vi "Ejercicio 2.1.vi"() -> ()   [LabVIEW 2021]
panel:
  out "[0.75 , 1]":dbl
  out "[0.5 , 0.75]":dbl
  out "[0.25 , 0.5]":dbl
  out "[0 , 0.25]":dbl
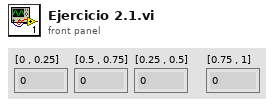
[diagram p1: front panel]
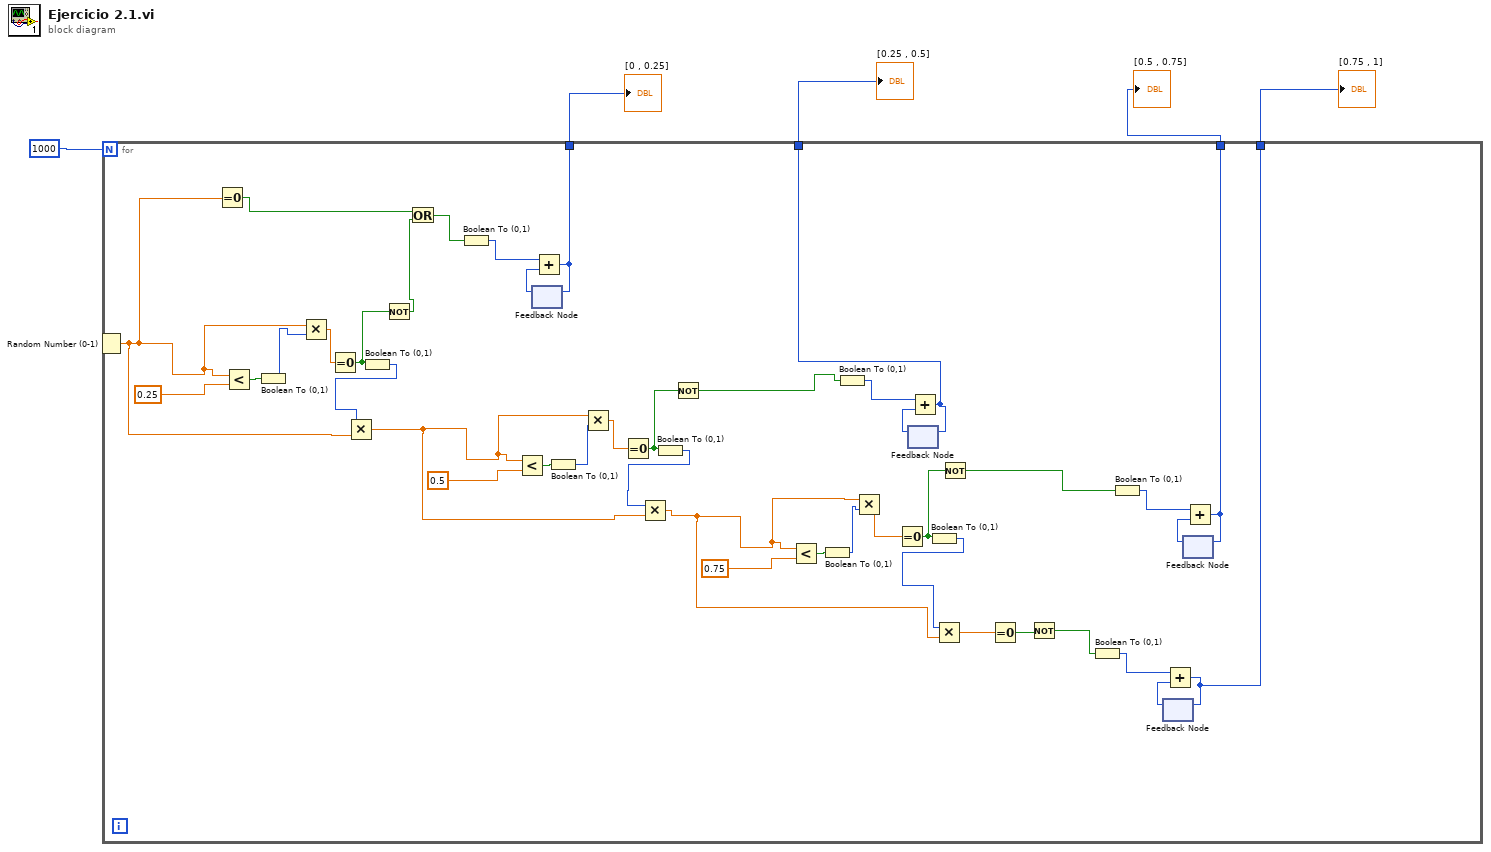
[diagram p0: block diagram]
diagram:
  n1 = for {
    N: 1000 -> [_]
    tunnel: [w18] -> w4
    tunnel: [w8] -> w3
    tunnel: [w7] -> w2
    tunnel: [w6] -> w1
    n2 = Random Number (0-1)() -> (number: 0 to 1=w24:dbl)
    n3 = Equal To 0?(x=w24) -> (x = 0?=w23:bool)
    n4 = Less?(x=w24, y=0.25) -> (x < y?=w46:bool)
    n5 = Boolean To (0,1)(Boolean=w46) -> (0, 1=w37:i16)
    n6 = Multiply(x=w24, y=w37) -> (x*y=w36:dbl)
    n7 = Equal To 0?(x=w36) -> (x = 0?=w41:bool)
    n8 = Boolean To (0,1)(Boolean=w41) -> (0, 1=w31:i16)
    n9 = Multiply(x=w31, y=w24) -> (x*y=w30:dbl)
    n10 = Not(x=w41) -> (.not. x?=w22:bool)
    n11 = Or(x=w23, y=w22) -> (x .or. y?=w21:bool)
    n12 = Boolean To (0,1)(Boolean=w21) -> (0, 1=w20:i16)
    n13 = Less?(x=w30, y=0.5) -> (x < y?=w44:bool)
    n14 = feedback #1() -> (w19:i16)  [unwired: 1 in]
    n15 = Add(x=w20, y=w19) -> (x+y=w18:i16)
    n16 = feedback-in #1(w18) -> ()
    n17 = Boolean To (0,1)(Boolean=w44) -> (0, 1=w35:i16)
    n18 = Multiply(x=w30, y=w35) -> (x*y=w34:dbl)
    n19 = Equal To 0?(x=w34) -> (x = 0?=w40:bool)
    n20 = Boolean To (0,1)(Boolean=w40) -> (0, 1=w29:i16)
    n21 = Multiply(x=w29, y=w30) -> (x*y=w27:dbl)
    n22 = Not(x=w40) -> (.not. x?=w9:bool)
    n23 = Less?(x=w27, y=0.75) -> (x < y?=w42:bool)
    n24 = Boolean To (0,1)(Boolean=w42) -> (0, 1=w33:i16)
    n25 = Boolean To (0,1)(Boolean=w9) -> (0, 1=w17:i16)
    n26 = Multiply(x=w27, y=w33) -> (x*y=w32:dbl)
    n27 = Equal To 0?(x=w32) -> (x = 0?=w39:bool)
    n28 = feedback #2() -> (w16:i16)  [unwired: 1 in]
    n29 = Add(x=w17, y=w16) -> (x+y=w8:i16)
    n30 = feedback-in #2(w8) -> ()
    n31 = Boolean To (0,1)(Boolean=w39) -> (0, 1=w28:i16)
    n32 = Multiply(x=w28, y=w27) -> (x*y=w26:dbl)
    n33 = Not(x=w39) -> (.not. x?=w10:bool)
    n34 = Equal To 0?(x=w26) -> (x = 0?=w25:bool)
    n35 = Not(x=w25) -> (.not. x?=w11:bool)
    n36 = Boolean To (0,1)(Boolean=w11) -> (0, 1=w13:i16)
    n37 = Boolean To (0,1)(Boolean=w10) -> (0, 1=w15:i16)
    n38 = feedback #3() -> (w12:i16)  [unwired: 1 in]
    n39 = Add(x=w13, y=w12) -> (x+y=w6:i16)
    n40 = feedback-in #3(w6) -> ()
    n41 = feedback #4() -> (w14:i16)  [unwired: 1 in]
    n42 = Add(x=w15, y=w14) -> (x+y=w7:i16)
    n43 = feedback-in #4(w7) -> ()
  }
  "[0 , 0.25]" <- w4
  "[0.25 , 0.5]" <- w3
  "[0.5 , 0.75]" <- w2
  "[0.75 , 1]" <- w1
